vi "Preferences UI.vi"() -> ()   [LabVIEW 2020, in "Performance Monitor UI.lvlib" / "Configuration.lvlib"]
doc: "Module UI that appears in the DCFG Framework for the Preferences View.\n_____\nBased on DCFG Project Template 1.0.0.21.\n____\nPeloton Config 1.0.0.2\nCopyright (c) 2022, Peloton"
uses:
  Configuration.lvlib
  <vilib>/Delacor/Delacor QMH/Libraries/Cloneable Module Admin_class/Delacor_lib_QMH_Cloneable Module Admin.lvclass
  Configuration--cluster.ctl
  <vilib>/Peloton/Peloton Config/Libraries/DCFG Page/Peloton_DCFG Page.lvlib
  <vilib>/Peloton/Pelobuttons/Pelobuttons_lib_Pelobuttons.lvlib
panel:
  in  "Random Path":path caption="Path"
  in  "Module Admin":refnum<class "Delacor_lib_QMH_Cloneable Module Admin.lvclass">
  in  "Values in":variant
  in  "Initialized":refnum<notifier>
  # "Note: Remember to use Pelobuttons for your UI"
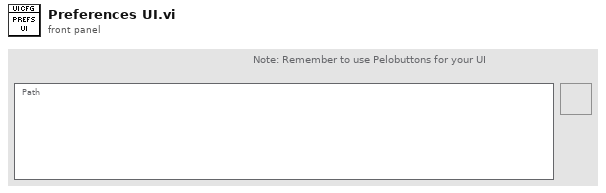
[diagram p1: front panel]
types:
  T1 = typedef "Performance Monitor UI.lvlib/Configuration.lvlib/Configuration--cluster.ctl" = cluster{"Random Path":path}
  T2 = enum32{"Invalid", "Standard", "Closed", "Hidden", "Minimized", "Maximized"}
  T3 = typedef "Peloton_DCFG Page.lvlib/Broadcast Events--cluster.ctl" = cluster{"Module Did Init":refnum<user-event>, "Status Updated":refnum<user-event>, "Error Reported":refnum<user-event>, "Module Did Stop":refnum<user-event>, "Send Data":refnum<user-event>, "Receive Data":refnum<user-event>, "Defaults Set":refnum<user-event>, "Update Module Execution Status":refnum<user-event>, "Unapplied Changes":refnum<user-event>}
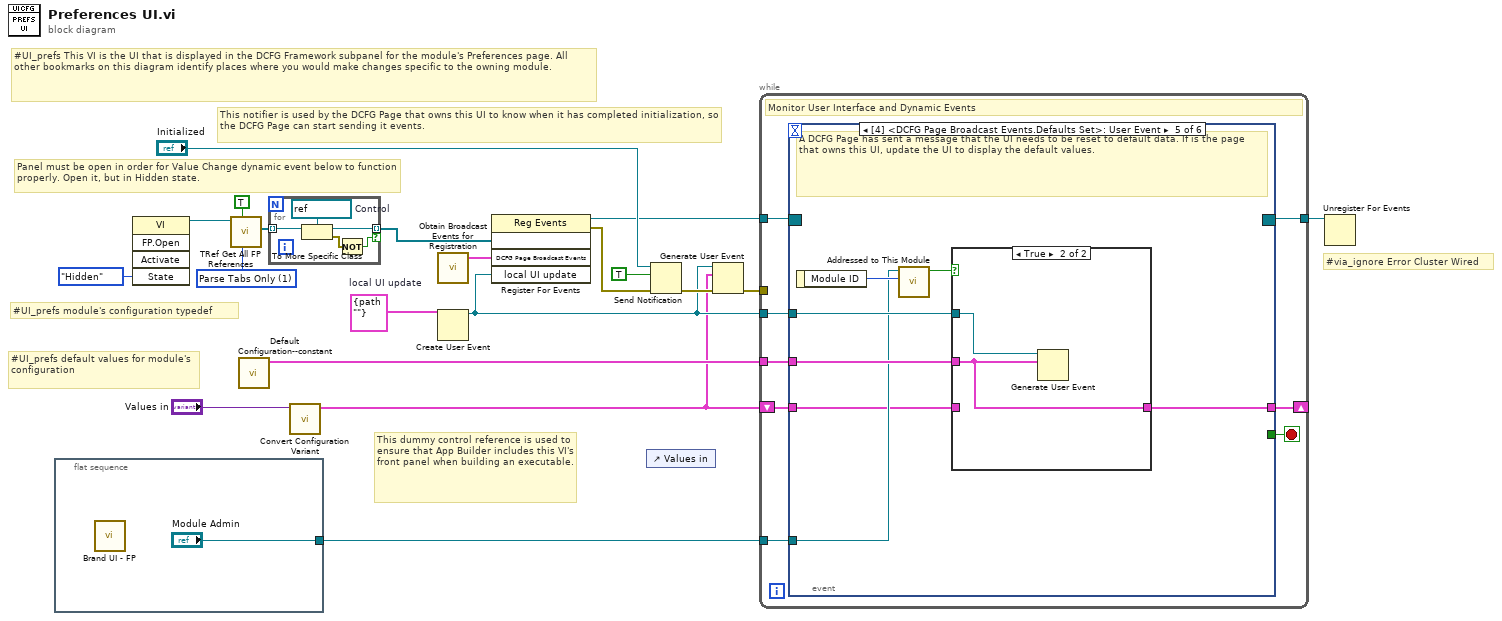
[diagram p0: block diagram]
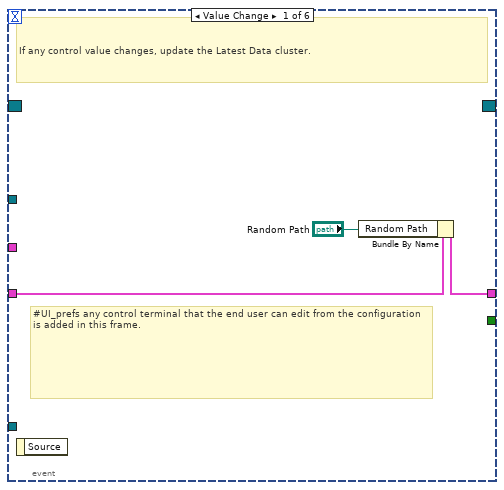
[diagram p2: hidden frame]
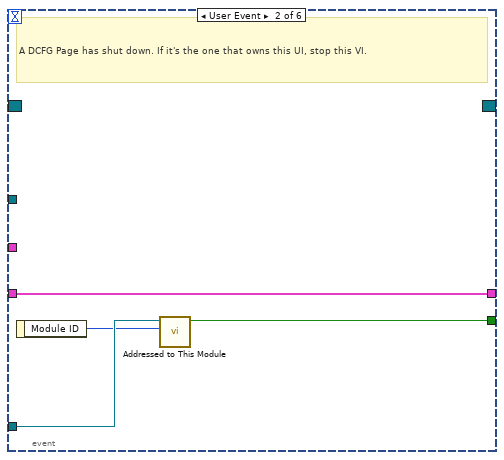
[diagram p3: hidden frame]
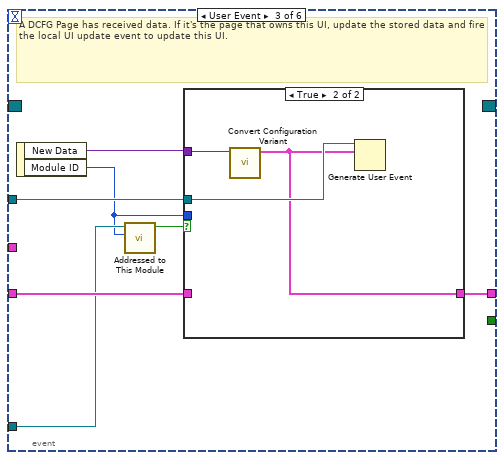
[diagram p4: hidden frame]
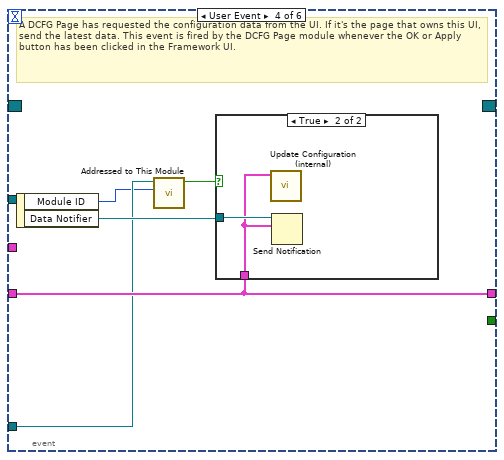
[diagram p6: hidden frame]
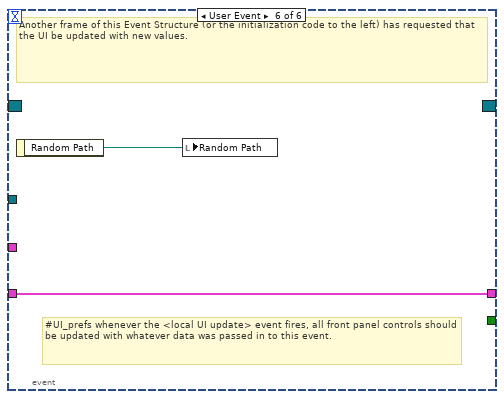
[diagram p9: hidden frame]
diagram:
  w3 = u16 1 items=["Parse All", "Parse Tabs Only"] ("Parsing Rule")
  w11 = T1 {"Random Path"=path ""}  # local UI update
  # "#via_ignore Error Cluster Wired"
  # "This dummy control reference is used to ensure that App Builder includes this VI's front panel when building an executable."
  # "Panel must be open in order for Value Change dynamic event below to function properly. Open it, but in Hidden state."
  # "This notifier is used by the DCFG Page that owns this UI to know when it has completed initialization, so the DCFG Page can start sending it events."
  # "#UI_prefs module's configuration typedef"
  # "#UI_prefs default values for module's configuration"
  # "#UI_prefs This VI is the UI that is displayed in the DCFG Framework subpanel for the module's Preferences page. All other bookmarks on this diagram identify places where you would make changes specific to the owning module."
  n1 = flat-sequence {
    tunnel: ["Module Admin"] -> w12
    frame #0 {
      n2 = call <vilib>:"Brand UI - FP.vi"() -> ()  [unwired: 12 in]
    }
  }
  n3 = invoke class="VI" method="FP.Open"("State"=T2."Hidden") -> (reference out=w5:refnum<vi>)  [unwired: 4 in, 4 out]
  n4 = call <vilib>:"TRef Get All FP References.vi"("Parsing Rule"=w3, "Ignore Decorations?"=TRUE, "VI Refnum"=w5) -> ("All FP Objects"=w2:refnum<vi>[])  [unwired: 4 in, 4 out]
  n5 = call "Default Configuration--constant.vi"() -> ("Default Configuration"=w8:T1)  [unwired: 11 in]
  n6 = for {
    tunnel: w2 -> [w26] mode=indexing
    tunnel: [w25] -> w1 mode=indexing if=w22
    w24 = refnum<vi> refnum  # Control
    n7 = To More Specific Class(target class=w24, reference=w26) -> (specific class reference=w25:refnum<vi>, error out=w23:errorcluster)  [unwired: 1 in]
    n8 = Not(x=w23) -> (.not. x?=w22:bool)
  }
  n9 = call "Convert Configuration Variant.vi"("Current Configuration"="Values in") -> ("Configuration"=w6:T1)  [unwired: 8 in, 2 out]
  n10 = call <vilib>:"Obtain Broadcast Events for Registration.vi"() -> ("DCFG Page Broadcast Events"=w19:T3)  [unwired: 9 in, 2 out]
  n11 = Create User Event(user event datatype=w11) -> (user event=w9:refnum<user-event>)  [unwired: 1 in, 1 out]
  n12 = register-events(w1, w19, w9) -> (reference out=w15:refnum<event-registration>, error out=w13:errorcluster)  [unwired: 2 in]
  n13 = control-ref of="Values in"() -> ()  [unwired: 1 out]
  n14 = Send Notification(notification=TRUE, notifier="Initialized", error in (no error)=w13) -> (error out=w16:errorcluster)  [unwired: 1 out]
  n15 = Generate User Event(user event=w9, event data cluster=w6, error in=w16) -> (error out=w10:errorcluster)  [unwired: 1 in, 1 out]
  n16 = while {
    tunnel: w10 -> [_]
    tunnel: w15 -> [w34]
    tunnel: [w33] -> w14
    shift-right: [w29] -> _
    shift-left: w6 -> [w32]
    tunnel: w12 -> [w30]
    tunnel: w8 -> [w28]
    tunnel: w9 -> [w27]
    stop <- w31 stop-if-true
    # "Monitor User Interface and Dynamic Events"
    n17 = event shown="[4] <DCFG Page Broadcast Events.Defaults Set>: User Event" {
      selector: w34 -> [_ _ _ _ _ _]
      dyn-events: [_ _ _ _ _ _] -> w33
      timeout: _ -> [_ _ _ _ _ _]
      tunnel: w32 -> [w37 w41 w48 w56 w61 w71]
      tunnel: [w36 w41 w47 w56 w60 w71] -> w29
      tunnel: [_ w38 _ _ _ _] -> w31
      tunnel: w30 -> [_ w40 w43 w55 w63 _]
      tunnel: w28 -> [_ _ _ _ w66 _]
      tunnel: w27 -> [_ _ w45 _ w65 _]
      event Value Change {
        # "#UI_prefs any control terminal that the end user can edit from the configuration is added in this frame."
        # "If any control value changes, update the Latest Data cluster."
        n18 = event-data() -> ()  [unwired: 1 in, 1 out]
        n19 = Bundle By Name(cluster=w37, "Random Path"="Random Path") -> (w36:T1)
      }
      event User Event {
        # "A DCFG Page has shut down. If it's the one that owns this UI, stop this VI."
        n20 = event-data() -> ("Module ID"=w39:i32)  [unwired: 1 in]
        n21 = call <vilib>:"Addressed to This Module.vi"("Module ID from Argument"=w39, "Module Admin"=w40) -> ("Addressed to this instance?"=w38:bool)  [unwired: 8 in, 1 out]
      }
      event User Event {
        # "A DCFG Page has received data. If it's the page that owns this UI, update the stored data and fire the local UI update event to update this UI."
        n22 = event-data() -> ("New Data"=w46:variant, "Module ID"=w42:i32)  [unwired: 1 in]
        n23 = call <vilib>:"Addressed to This Module.vi"("Module ID from Argument"=w42, "Module Admin"=w43) -> ("Addressed to this instance?"=w44:bool)  [unwired: 8 in, 1 out]
        n24 = case shown="True" w44 {
          tunnel: w48 -> [w49 _]
          tunnel: [w49 w50] -> w47
          tunnel: w46 -> [_ w51]
          tunnel: w45 -> [_ w52]
          tunnel: w42 -> [_ _]
          frame False {
          }
          frame True {
            n25 = call "Convert Configuration Variant.vi"("Current Configuration"=w51) -> ("Configuration"=w50:T1)  [unwired: 8 in, 2 out]
            n26 = Generate User Event(user event=w52, event data cluster=w50) -> ()  [unwired: 2 in, 2 out]
          }
        }
      }
      event User Event {
        # "A DCFG Page has requested the configuration data from the UI. If it's the page that owns this UI, send the latest data. This event is fired by the DCFG Page module whenever the OK or Apply button has been clicked in the Framework UI."
        n27 = event-data() -> ("Module ID"=w53:i32, "Data Notifier"=w57:refnum<notifier>)  [unwired: 1 in]
        n28 = call <vilib>:"Addressed to This Module.vi"("Module ID from Argument"=w53, "Module Admin"=w55) -> ("Addressed to this instance?"=w54:bool)  [unwired: 8 in, 1 out]
        n29 = case shown="True" w54 {
          tunnel: w57 -> [_ w59]
          tunnel: w56 -> [_ w58]
          frame False {
          }
          frame True {
            n30 = call "Update Configuration (internal).vi"("configuration"=w58) -> ()  [unwired: 11 in]
            n31 = Send Notification(notification=w58, notifier=w59) -> ()  [unwired: 1 in, 2 out]
          }
        }
      }
      event User Event {
        # "A DCFG Page has sent a message that the UI needs to be reset to default data. If is the page that owns this UI, update the UI to display the default values."
        n32 = event-data() -> ("Module ID"=w64:i32)  [unwired: 1 in]
        n33 = call <vilib>:"Addressed to This Module.vi"("Module ID from Argument"=w64, "Module Admin"=w63) -> ("Addressed to this instance?"=w62:bool)  [unwired: 8 in, 1 out]
        n34 = case shown="True" w62 {
          tunnel: w66 -> [_ w68]
          tunnel: w65 -> [_ w69]
          tunnel: w61 -> [w67 _]
          tunnel: [w67 w68] -> w60
          frame False {
          }
          frame True {
            n35 = Generate User Event(user event=w69, event data cluster=w68) -> ()  [unwired: 2 in, 2 out]
          }
        }
      }
      event User Event {
        # "#UI_prefs whenever the <local UI update> event fires, all front panel controls should be updated with whatever data was passed in to this event."
        # "Another frame of this Event Structure (or the initialization code to the left) has requested that the UI be updated with new values."
        n36 = event-data() -> ("Random Path"=w70:path)  [unwired: 1 in]
        n37 = local write "Random Path"(w70) -> ()
      }
    }
  }
  n38 = Unregister For Events(event registration refnum=w14) -> ()  [unwired: 1 in, 1 out]
